vi "曲线去两端.vi"(11 "曲线In":cluster{"X":dbl[], "Y":dbl[]}[](array[cluster])) -> (2 "启动曲线":cluster{"X":dbl[], "Y":dbl[]}[](array[cluster]), 3 "曲线Out":cluster{"X":dbl[], "Y":dbl[]}[](array[cluster]))   [LabVIEW 2020]
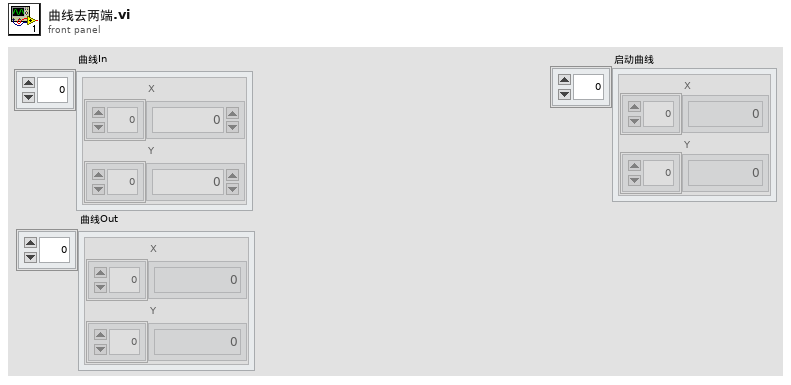
[diagram p1: front panel]
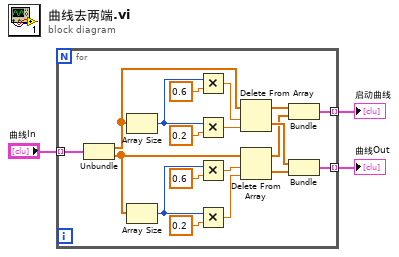
[diagram p0: block diagram]
diagram:
  n1 = for {
    tunnel: "曲线In" -> [w19] mode=indexing
    tunnel: [w11] -> w2 mode=indexing
    tunnel: [w7] -> w1 mode=indexing
    n2 = Unbundle(w19) -> ("X"=w15:dbl[], "Y"=w13:dbl[])
    n3 = Array Size(array=w15) -> (size(s)=w21:i32)
    n4 = Array Size(array=w13) -> (size(s)=w17:i32)
    n5 = Multiply(x=w21, y=0.6) -> (x*y=w10:dbl)
    n6 = Multiply(x=w21, y=0.2) -> (x*y=w9:dbl)
    n7 = Multiply(x=w17, y=0.6) -> (x*y=w5:dbl)
    n8 = Multiply(x=w17, y=0.2) -> (x*y=w6:dbl)
    n9 = Delete From Array(array=w15, length=w10, index=w9) -> (deleted portion=w14:dbl[], array with subset deleted=w8:dbl[])
    n10 = Delete From Array(array=w13, length=w5, index=w6) -> (deleted portion=w12:dbl[], array with subset deleted=w4:dbl[])
    n11 = Bundle("X"=w8, "Y"=w4) -> (w7:cluster{"X":dbl[], "Y":dbl[]})  [unwired: 1 in]
    n12 = Bundle("X"=w14, "Y"=w12) -> (w11:cluster{"X":dbl[], "Y":dbl[]})  [unwired: 1 in]
  }
  "曲线Out" <- w2
  "启动曲线" <- w1
